vi "Photon Counter SR400.vi"(8 "error in (no error)":errorcluster) -> (0 "error out":errorcluster, 3 "Photon Counter SR400 out":refnum<class "Photon Counter SR400.lvclass">)   [LabVIEW 2009, in "Photon Counter SR400.lvclass"]
uses:
  Photon Counter SR400.lvclass
  Global/GPIB Numbers.vi
  Utility Classes/Readable/Readable.lvclass
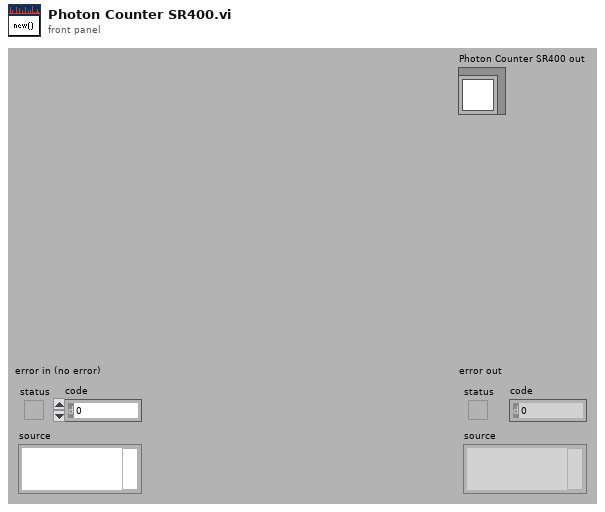
[diagram p1: front panel]
types:
  T1 = typedef "GPIB Type Def.ctl" = cluster{"Name":string, "bus":dbl, "GPIB":dbl, "GPIB as string":string, "byte":i32, "VISA Resource Name":refnum<visa-resource-name>}
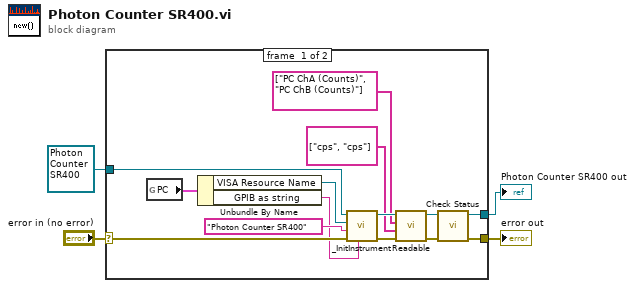
[diagram p0: block diagram]
diagram:
  n1 = case shown="No Error" "error in (no error)" {
    selector: "error in (no error)" -> [w17 w20]
    tunnel: [w10 w20] -> w3
    tunnel: [w11 w19] -> w2
    tunnel: refnum<class "Photon Counter SR400.lvclass"> refnum ("Photon Counter SR400.lvclass") -> [w18 w19]
    frame #0 {
      n2 = global read "GPIB Numbers.vi" "PC"() -> (w15:T1)
      n3 = Unbundle By Name(w15) -> ("VISA Resource Name"=w14:refnum<visa-resource-name>, "GPIB as string"=w13:string)
      n4 = call-dynamic "_InitInstrument.vi"("GPIB as string"=w13, "error in (no error)"=w17, "Name"="Photon Counter SR400", "VISA Resource Name"=w14, "Instrument in"=w18) -> ("error out"=w6:errorcluster, "Instrument out"=w12:refnum<class "Photon Counter SR400.lvclass">)  [unwired: 1 in, 4 out]
      n5 = call "Readable.vi"("error in (no error)"=w6, "Channel Units"=string[] ["cps", "cps"], "Channel Names"=string[] ["PC ChA (Counts)", "PC ChB (Counts)"], "Readable in"=w12) -> ("error out"=w5:errorcluster, "Readable out"=w9:refnum<class "Photon Counter SR400.lvclass">)  [unwired: 6 in]
      n6 = call-dynamic "Check Status.vi"("error in (no error)"=w5, "Photon Counter SR400 in"=w9) -> ("error out"=w10:errorcluster, "Photon Counter SR400 out"=w11:refnum<class "Photon Counter SR400.lvclass">)  [unwired: 8 out]
    }
    frame #1 {
    }
  }
  "error out" <- w3
  "Photon Counter SR400 out" <- w2
